vi "Drive Data Logger.vi"(5 "Save":bool, 6 "Array":dbl[](array[numeric]), 7 "Burst":i32, 10 "rt fifo":refnum<k33>, 11 "TDMS Refnum":refnum<k34>) -> ()   [LabVIEW 2013]
panel:
  in  "rt fifo 2":refnum<k33>
  in  "Array 4":i32[](array[numeric])
  in  "Array 3":i32[](array[numeric])
  out "error out 2":errorcluster
  in  "Refnum in 2":refnum<k34>
  out "# elements 2":u32
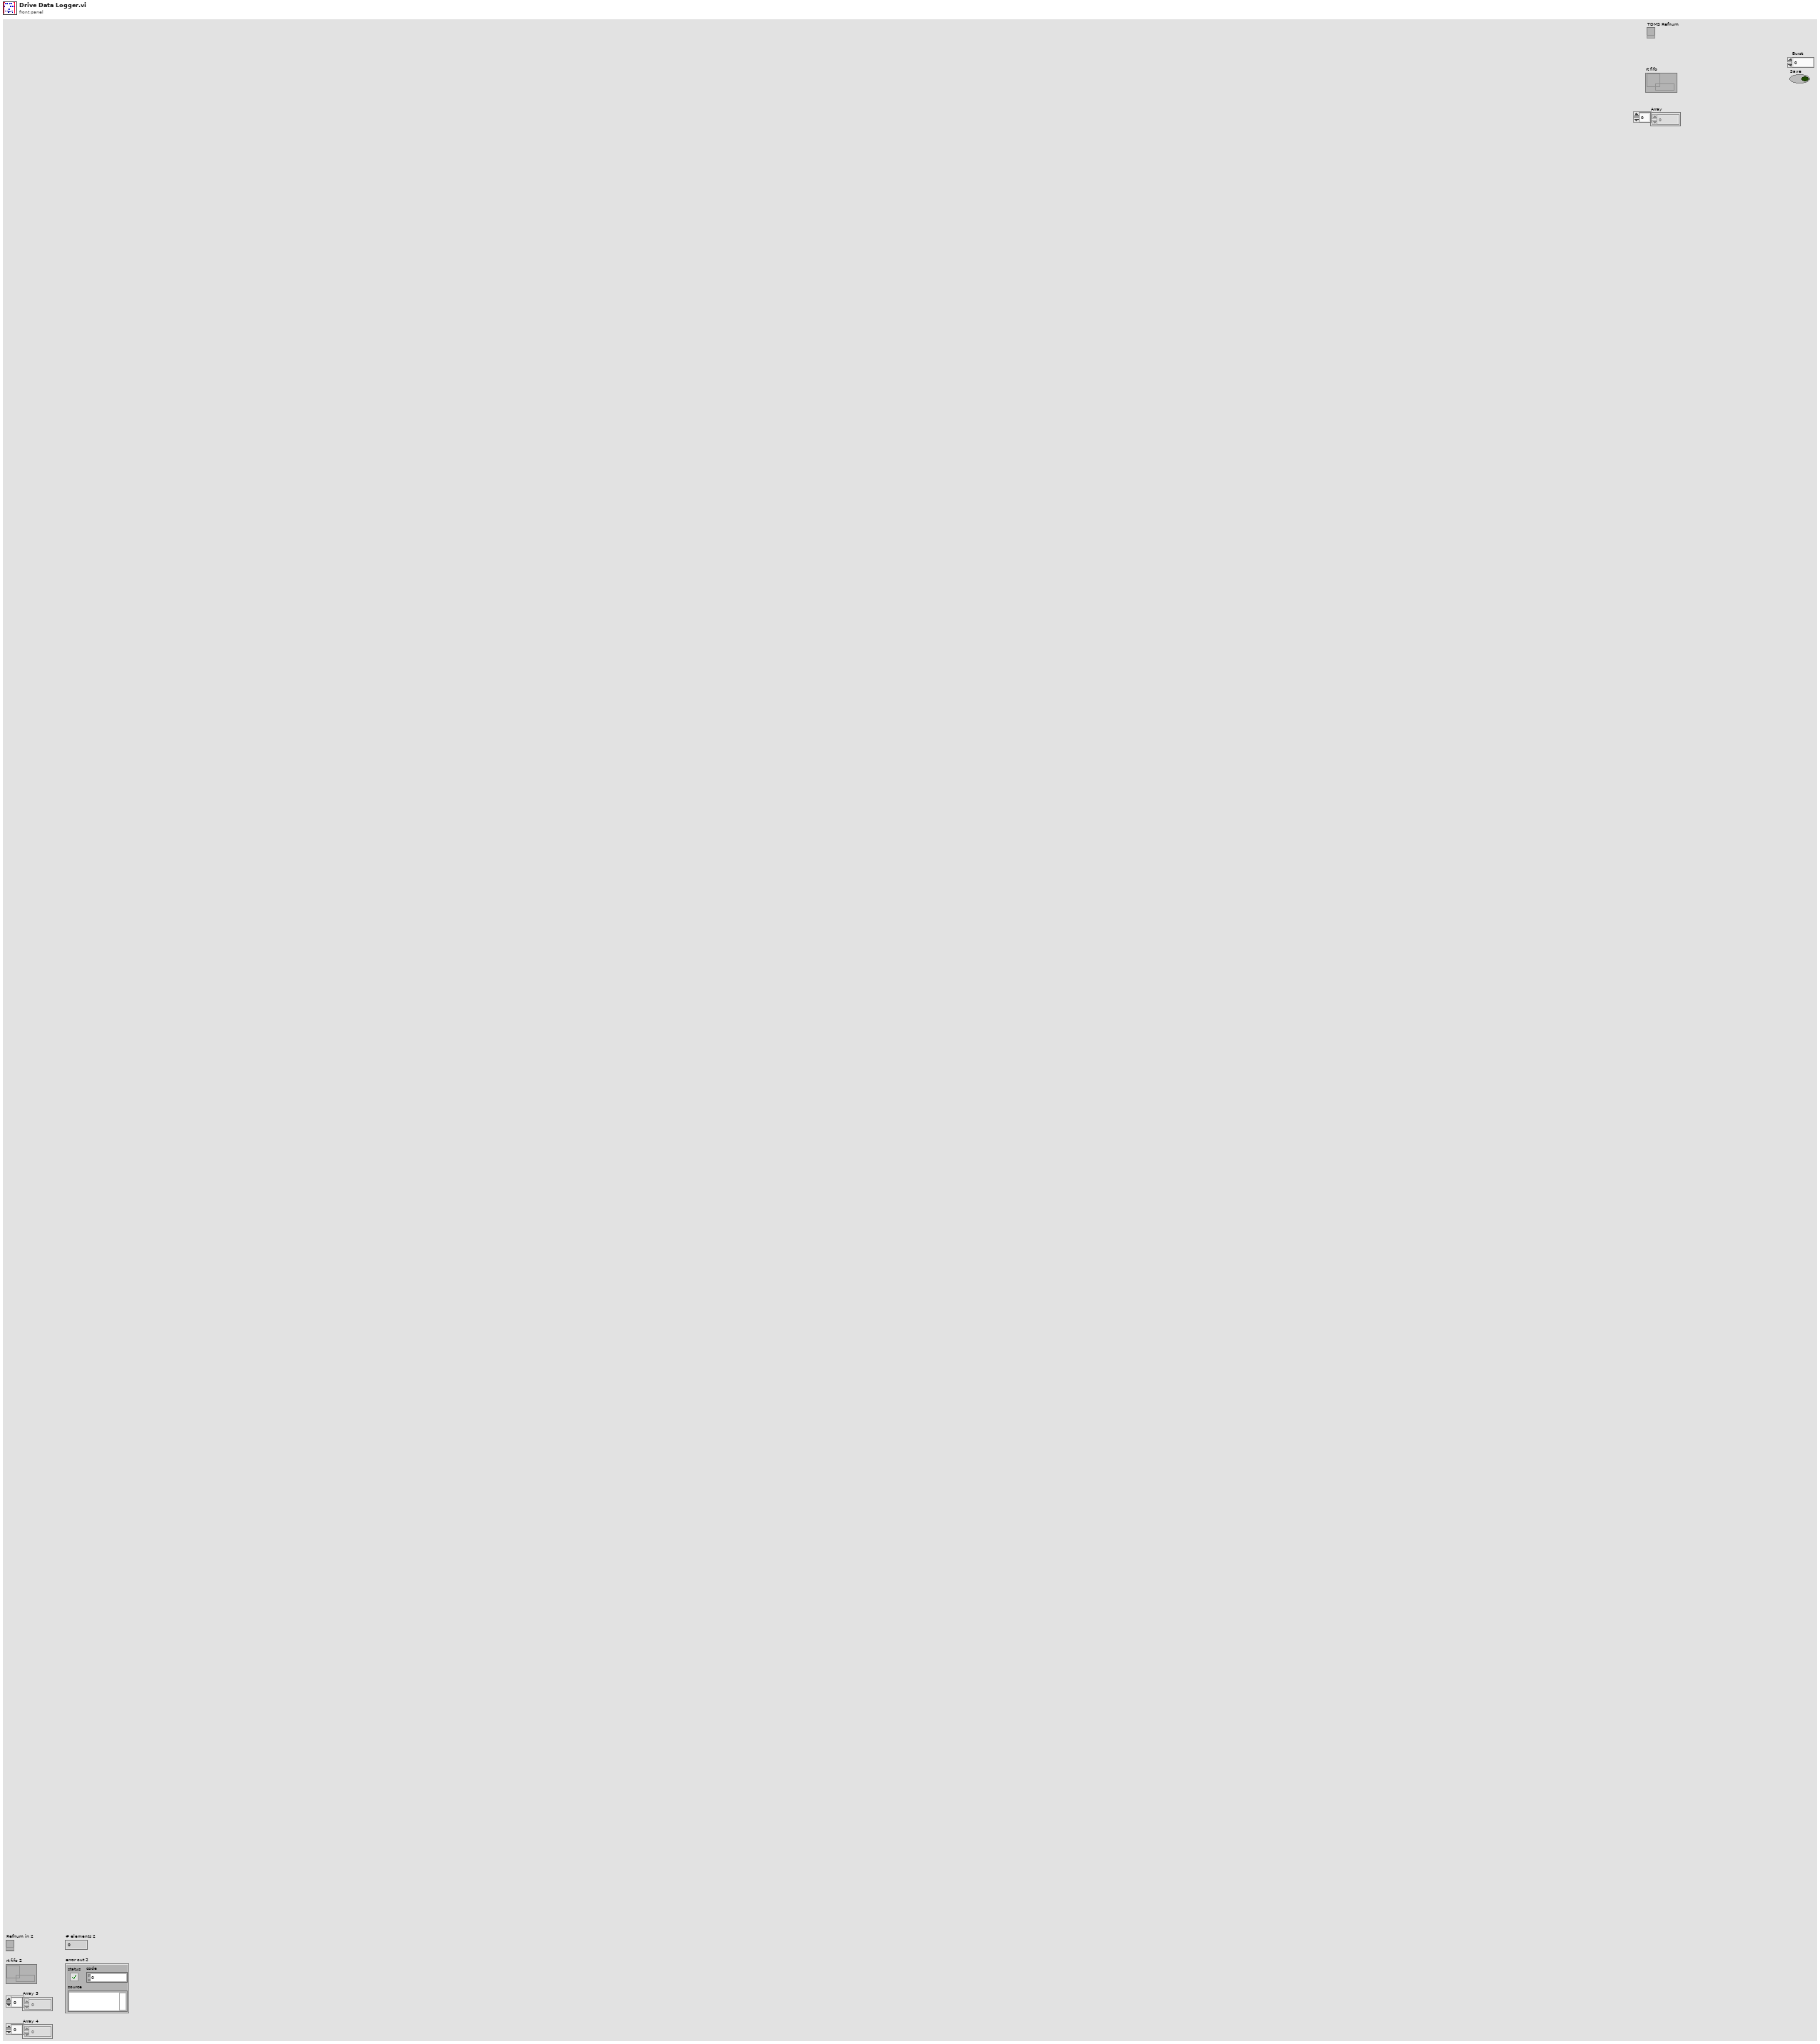
[diagram p1: front panel]
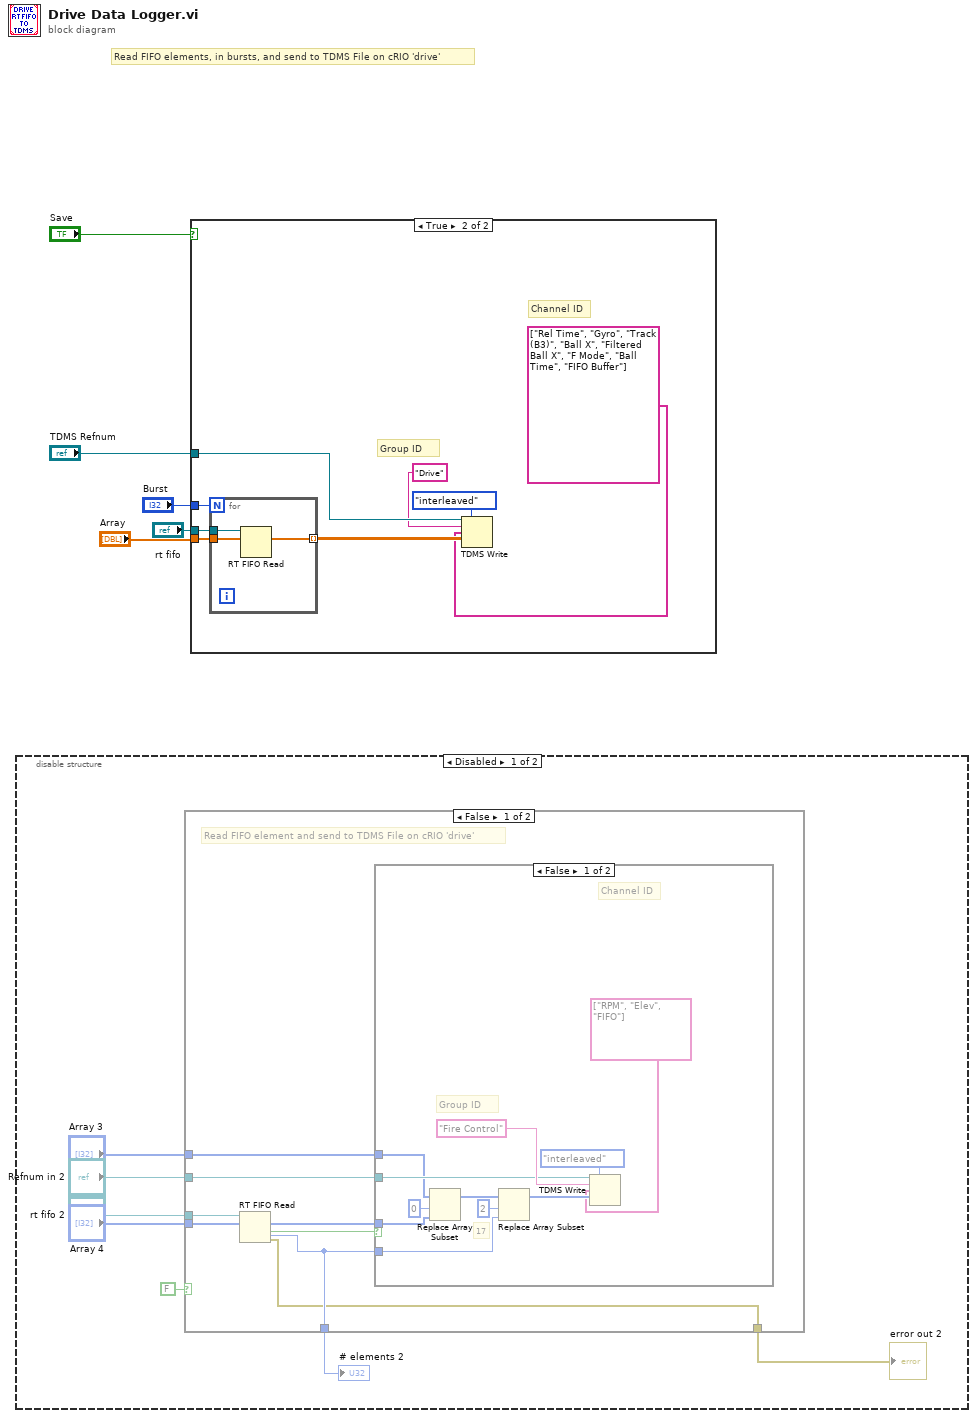
[diagram p0: block diagram]
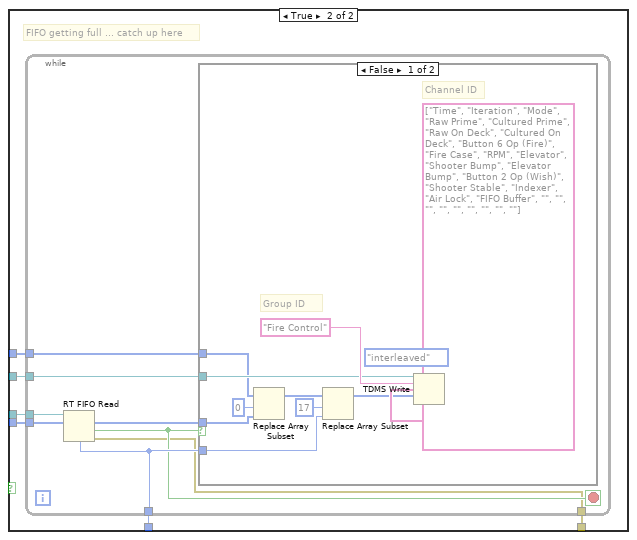
[diagram p4: hidden frame]
diagram:
  # "Read FIFO elements, in bursts, and send to TDMS File on cRIO 'drive'"
  n1 = disable-structure shown="Disabled" {
    frame Disabled {
      n2 = case shown="False" FALSE {
        tunnel: "rt fifo 2" -> [w20 w37]
        tunnel: "Refnum in 2" -> [w17 w36]
        tunnel: "Array 4" -> [w16 w35]
        tunnel: "Array 3" -> [w15 w34]
        tunnel: [w14 w33] -> w12
        tunnel: [w13 w32] -> w9
        frame False {
          # "Read FIFO element and send to TDMS File on cRIO 'drive'"
          n3 = RT FIFO Read(0:w20, 1:w16) -> (7:w14:u32, 9:w19:i32[], 10:w18:bool, 11:w13:errorcluster)  [unwired: 2 in, 1 out]
          n4 = case shown="False" w18 {
            tunnel: w19 -> [w28 _]
            tunnel: w17 -> [w30 _]
            tunnel: w15 -> [w27 _]
            tunnel: w14 -> [w24 _]
            frame False {
              # "17"
              # "Group ID"
              # "Channel ID"
              n5 = Replace Array Subset(array=w27, new element=w28, index=0) -> (w26:i32[])
              n6 = Replace Array Subset(array=w26, new element=w24, index=2) -> (w23:i32[])
              n7 = TDMS Write(0:w30, 1:enum16{"decimated", "interleaved"}."interleaved" ("data layout (0:decimated)"), 5:"Fire Control" ("group name in (Untitled)"), 7:string[] ["RPM", "Elev", "FIFO"] ("channel name(s) in (Untitled)"), 9:w23) -> ()  [unwired: 1 in, 4 out]
            }
            frame True {
              # "No data in FIFO to log"
            }
          }
        }
        frame True {
          # "FIFO getting full ... catch up here"
          n8 = while {
            tunnel: w37 -> [w45]
            tunnel: w36 -> [w43]
            tunnel: w35 -> [w42]
            tunnel: w34 -> [w41]
            tunnel: [w40] -> w33
            tunnel: [w38] -> w32
            stop <- w39 stop-if-true
            n9 = RT FIFO Read(0:w45, 1:w42) -> (7:w40:u32, 9:w44:i32[], 10:w39:bool, 11:w38:errorcluster)  [unwired: 2 in, 1 out]
            n10 = case shown="False" w39 {
              tunnel: w44 -> [w51 _]
              tunnel: w43 -> [w53 _]
              tunnel: w41 -> [w50 _]
              tunnel: w40 -> [w47 _]
              frame False {
                # "Group ID"
                # "Channel ID"
                n11 = Replace Array Subset(array=w50, new element=w51, index=0) -> (w49:i32[])
                n12 = Replace Array Subset(array=w49, new element=w47, index=17) -> (w46:i32[])
                n13 = TDMS Write(0:w53, 1:enum16{"decimated", "interleaved"}."interleaved" ("data layout (0:decimated)"), 5:"Fire Control" ("group name in (Untitled)"), 7:string[] ["Time", "Iteration", "Mode", "Raw Prime", "Cultured Prime", "Raw On Deck", "Cultured On Deck", "Button 6 Op (Fire)", "Fire Case", "RPM", "Elevator", "Shooter Bump", "Elevator Bump", "Button 2 Op (Wish)", "Shooter Stable", "Indexer", "Air Lock", "FIFO Buffer", "", "", "", "", "", "", "", "", ""] ("channel name(s) in (Untitled)"), 9:w46) -> ()  [unwired: 1 in, 4 out]
              }
              frame True {
                # "No data in FIFO to log"
              }
            }
          }
        }
      }
      "# elements 2" <- w12
      "error out 2" <- w9
    }
    frame Enabled {
    }
  }
  n14 = case shown="True" "Save" {
    tunnel: "rt fifo" -> [_ w64]
    tunnel: "TDMS Refnum" -> [_ w63]
    tunnel: "Array" -> [_ w62]
    tunnel: "Burst" -> [_ w58]
    frame False {
    }
    frame True {
      # "Channel ID"
      # "Group ID"
      n15 = for {
        N: w58 -> [_]
        tunnel: w64 -> [w67]
        tunnel: [w66] -> w59 mode=indexing
        tunnel: w62 -> [w65]
        n16 = RT FIFO Read(0:w67, 1:w65) -> (9:w66:dbl[])  [unwired: 2 in, 4 out]
      }
      n17 = TDMS Write(0:w63, 1:enum16{"decimated", "interleaved"}."interleaved" ("data layout (0:decimated)"), 5:"Drive" ("group name in (Untitled)"), 7:string[] ["Rel Time", "Gyro", "Track (B3)", "Ball X", "Filtered Ball X", "F Mode", "Ball Time", "FIFO Buffer"] ("channel name(s) in (Untitled)"), 9:w59) -> ()  [unwired: 1 in, 4 out]
    }
  }
